vi "PassiveAggressiveRegressor.vi"(8 "error in":errorcluster) -> (0 "error out":errorcluster, 3 "out":refnum<class "PassiveAggressiveRegressor.lvclass">)   [LabVIEW 2020]
doc: "Passive Aggressive Regressor\n\n Read more in the :ref:`User Guide <passive_aggressive>`.\n\n Parameters\n ----------\n\n C : float, default=1.0\n Maximum step size (regularization). Defaults to 1.0.\n\n fit_intercept : bool, default=True\n Whether the intercept should be estimated or not. If False, the\n data is assumed to be already centered. Defaults to True.\n\n max_iter : int, default=1000\n The maximum number of passes over the training data (aka epochs).\n It only impacts the behavior in the ``fit`` method, and not the\n :meth:`partial_fit` method.\n\n .. versionadded:: 0.19\n\n tol : float or None, default=1e-3\n The stopping criterion. If it is not None, the iterations will stop\n when (loss > previous_loss - tol).\n\n .. versionadded:: 0.19\n\n early_stopping : bool, default=False\n Whether to use early stopping to terminate training when validation.\n score is not improving. If set to True, it will automatically set aside\n a fraction of training data as validation and terminate\n training when validation score is not improving by at least tol for\n n_iter_no_change consecutive epochs.\n\n .. versionadded:: 0.20\n\n validation_fraction : float, default=0.1\n The proportion of training data to set aside as validation set for\n early stopping. Must be between 0 and 1.\n Only used if early_stopping is True.\n\n .. versionadded:: 0.20\n\n n_iter_no_change : int, default=5\n Number of iterations with no improvement to wait before early stopping.\n\n .. versionadded:: 0.20\n\n shuffle : bool, default=True\n Whether or not the training data should be shuffled after each epoch.\n\n verbose : integer, default=0\n The verbosity level\n\n loss : string, default=\"epsilon_insensitive\"\n The loss function to be used:\n epsilon_insensitive: equivalent to PA-I in the reference paper.\n squared_epsilon_insensitive: equivalent to PA-II in the reference\n paper.\n\n epsilon : float, default=0.1\n If the difference between the current prediction and the correct label\n is below this threshold, the model is not updated.\n\n random_state : int, RandomState instance, default=None\n Used to shuffle the training data, when ``shuffle`` is set to\n ``True``. Pass an int for reproducible output across multiple\n function calls.\n See :term:`Glossary <random_state>`.\n\n warm_start : bool, default=False\n When set to True, reuse the solution of the previous call to fit as\n initialization, otherwise, just erase the previous solution.\n See :term:`the Glossary <warm_start>`.\n\n Repeatedly calling fit or partial_fit when warm_start is True can\n result in a different solution than when calling fit a single time\n because of the way the data is shuffled.\n\n average : bool or int, default=False\n When set to True, computes the averaged SGD weights and stores the\n result in the ``coef_`` attribute. If set to an int greater than 1,\n averaging will begin once the total number of samples seen reaches\n average. So average=10 will begin averaging after seeing 10 samples.\n\n .. versionadded:: 0.19\n parameter *average* to use weights averaging in SGD\n\n Attributes\n ----------\n coef_ : array, shape = [1, n_features] if n_classes == 2 else [n_classes, n_features]\n Weights assigned to the features.\n\n intercept_ : array, shape = [1] if n_classes == 2 else [n_classes]\n Constants in decision function.\n\n n_iter_ : int\n The actual number of iterations to reach the stopping criterion.\n\n t_ : int\n Number of weight updates performed during training.\n Same as ``(n_iter_ * n_samples)``.\n\n \nAvailable methods:\nGet Attributes\nGet Params\nSet Params"
uses:
  PassiveAggressiveRegressor.lvclass
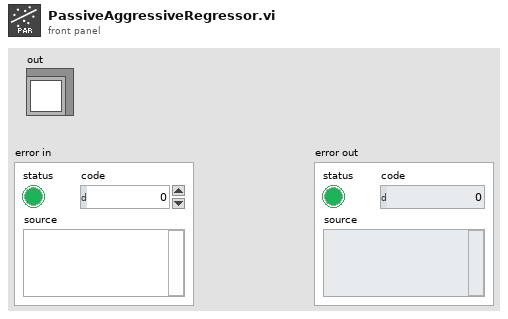
[diagram p1: front panel]
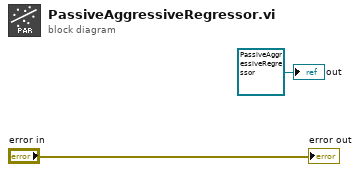
[diagram p0: block diagram]
diagram:
  "out" <- refnum<class "PassiveAggressiveRegressor.lvclass"> refnum ("model")
  "error out" <- "error in"
